vi "20210518_00_ATA_FPGA.vi"() -> ()   [LabVIEW 2018]
doc: "This FPGA VI transfers data samples to the host using a stream. The stream is controlled from the host."
uses:
  FPGA_Controls/FPGA_Enable_Clust.ctl
  FPGA_Controls/FPGA_Scale_Clust.ctl
  FPGA_Controls/FPGA_Probe_Clust.ctl
  <vilib>/Platform/TimedLoop/XDataNode/timing_clust.ctl
  <vilib>/Platform/TimedLoop/XDataNode/nitl_modes.ctl
  <vilib>/Platform/TimedLoop/XDataNode/wakeup.ctl
  FPGA_Controls/FilterStageEnum.ctl
  FPGA_Controls/FPGA_Shift_Enable.ctl
  <vilib>/rvi/Analysis/measure/FFT/simModelSupport/niFPGA FFT Outside SCTL Sim Properties.ctl
  <vilib>/rvi/Analysis/measure/FFT/simModelSupport/niFPGA FFT Sim Types.ctl
  <vilib>/rvi/Analysis/measure/FFT/simModelSupport/niFpgaFFTSimArithmeticProperties.ctl
  <vilib>/rvi/Analysis/measure/FFT/simModelSupport/niFpgaFFTSimDfxp.ctl
  <vilib>/fxp/LVFixedPointQuantizationPolicyTypeDef.ctl
  <vilib>/rvi/Emulation/niFpgaGetClockAttributes.vi
  <vilib>/rvi/Emulation/niFpgaSctlEmulationGetInTimedLoop.vi
  <vilib>/rvi/Emulation/niFpgaEmulationReportErrorSimple.vi
  <vilib>/rvi/eio/common/nirviEmuTemplateMethod_errors.vi
  <vilib>/rvi/Emulation/niFpgaCriticalErrorInLSC.vi
  <vilib>/rvi/DataTransferAndStorage/Container/Common/niFpgaContainerGetUniqueNameForEmu.vi
  <vilib>/rvi/DataTransferAndStorage/Container/Common/niFpgaContainerSetEmuInfo.vi
  <vilib>/rvi/eio/common/nirviEmuReportErrorAndStop.vi
  <vilib>/rvi/DataTransferAndStorage/Container/Common/niFpgaContainerExecOnDevCompGetState.vi
  <vilib>/rvi/Emulation/niFpgaEmulationIsFPGAContextNoSignature.vi
  <vilib>/rvi/Emulation/niFpgaProcessEmulError.vi
  <vilib>/rvi/errors/nirviReportUnexpectedCaseInternalError (U32).vi
  <vilib>/rvi/Memory/Memory_Emulation/niFpgaMemoryEmulationCacheClearOnFirstRun.vi
  <vilib>/rvi/Memory/Memory_Emulation/nirvimemoryEmulationManagerCache_MakeExclusive.vi
  <vilib>/rvi/Memory/Memory_Emulation/niFpgaMemoryEmulationValidateCache.vi
  <vilib>/rvi/Memory/Memory_Emulation/nirvimemoryEmulationManagerCache_InsertValue.vi
  <vilib>/Utility/error.llb/Clear Errors.vi
  <vilib>/rvi/Memory/Memory_Emulation/nirvimemoryEmulationManagerCache_ReleaseExclusive.vi
  <vilib>/rvi/Memory/Memory_Emulation/nirvimemoryEmulationManagerCache_GetValue.vi
  <vilib>/rvi/Memory/Memory_Emulation/nirvimemoryEmulationManagerCache_SetValue.vi
  <vilib>/rvi/Emulation/niFpgaSctlEmulationResourceMgr.vi
  <vilib>/rvi/errors/niFpgaSetErrorForExecOnDevCompSimple.vi
  <vilib>/rvi/FIFO/Fifo_Resource/nirvififoEmulationSetSize.vi
  <vilib>/rvi/FIFO/Fifo_Resource/nirviFifoEmulationQueueMgr.vi
  <instcachedir>/0/nirviFifoEmulationQueueMgr_E5CAEC123FF24DC58D834DCA3CDAA9B5.lvgen/nirviFifoEmulationQueueMgr_E5CAEC123FF24DC58D834DCA3CDAA9B5_000.vi
  <vilib>/rvi/FIFO/Fifo_Resource/nirvififoEmulationCreateLock.vi
  <vilib>/rvi/FIFO/Fifo_Resource/nirvififoEmulationObtainLock.vi
  <vilib>/rvi/FIFO/Fifo_Resource/nirvififoEmulationReleaseLock.vi
  <vilib>/rvi/occurrence/nirviWaitOnOccurrenceBase.vi
  <vilib>/rvi/errors/nirviReportUnexpectedCaseInternalError.vi
  <vilib>/rvi/Analysis/measure/FFT/simModelSupport/niFpgaFFTSimModelOutsideSCTLCore.vi
  <instrlib>/_niInstr/Basic Elements/v1/FPGA/Private/Count Up U16.vi
  <vilib>/rvi/interface/RandomDataEmulation/nirviRandomDataMultiElementFPGAFIFO.vi
  <instcachedir>/0/nirviRandomDataMultiElementFPGAFIFO_6740B454F3C245F78F76ED91F73FD8DB.lvgen/nirviRandomDataMultiElementFPGAFIFO_6740B454F3C245F78F76ED91F73FD8DB_001.vi
  <vilib>/rvi/interface/RandomDataEmulation/niFpgaRandomDataHandleErrors.vi
  <instrlib>/_niInstr/Basic Elements/v1/FPGA/Private/Count Up U32.vi
  <vilib>/rvi/FIFO/Fifo_Resource/nirvififoEmulationDetermineInputValidOut.vi
  <instrlib>/_niInstr/Basic Elements/v1/FPGA/Private/Count Up U8.vi
  <instcachedir>/0/nirviRandomDataMultiElementFPGAFIFO_6740B454F3C245F78F76ED91F73FD8DB.lvgen/nirviRandomDataMultiElementFPGAFIFO_6740B454F3C245F78F76ED91F73FD8DB_000.vi
  <vilib>/eio/EIONode/EIONode.xnode
  <vilib>/Platform/TimedLoop/XDataNode/XDataNode.xnode
  <vilib>/rvi/LocalResourceManager/LocalResourceManager.xnode
  <vilib>/rvi/DataTransferAndStorage/Container/XNode/niFpgaContainer.xnode
  <vilib>/rvi/Memory/Memory_Emulation/niFpgaMemoryEmulationRefIn.vi
  <vilib>/rvi/FIFO/Fifo_Resource/nirvififoEmulationRead.vi
  <vilib>/rvi/Analysis/measure/FFT/XNode/niFpgaFFT.xnode
  <vilib>/rvi/FXPMathLib/FxpMul/XNode/nifxpmath_Multiplier.xnode
  <vilib>/rvi/FXPMathLib/FxpAdd/XNode/nifxpmath_Add.xnode
  <vilib>/rvi/interface/RandomDataEmulation/nirviRandomDataFpgaMultiElementTemplate.vi
  <vilib>/rvi/FXPMathLib/FxpInterpret/XNode/nifxpmath_Interpret.xnode
  <vilib>/rvi/FIFO/Fifo_Resource/niFpgaFifoEmulationRefIn.vi
  <vilib>/Platform/TimedLoop/XDataNode/XDNodeRunTimeDep.lvlib
  <instrlib>/_niInstr/Basic Elements/v1/FPGA/niInstr Basic Elements v1 FPGA.lvlib
  <vilib>/rvi/FXPMathLib/sim/FxpSim.dll
panel:
  out "5_Seconds_Elapsed":bool
  in  "AllData_EvenInvalid":bool
  out "ValidPostShift":bool
  out "ValidPreShift":bool
  out "ValidScaleMeas":bool
  out "WritingToFIFO?":bool
  out "AI0_Unshifted_Index":u32
  out "AI0_Co_Beac_Q_Index":fxp<+/-,24,1>
  out "AI0_Co_I_Index":fxp<+/-,24,1>
  out "MaxMeas":fxp<+/-,24,1>
  in  "Ramp?":bool
  out "AI1_Over":bool
  out "AI0_Over":bool
  in  "Simulate?":bool
  out "Chan1_Beac_QProbe":T1
  out "Chan1_Beac_IProbe":T1
  out "Chan1_Cal_QProbe":T1
  out "Chan0_Beac_QProbe":T1
  out "Chan0_Beac_IProbe":T1
  out "Chan0_Cal_QProbe":T1
  out "NoiseFloorFFT_LoopCount 2":i32
  out "ReceiverTimed Out 2":bool
  out "SuccessiveIndeces 2":u16[](array[numeric])
  in  "#Avg 2":u16=1
  in  "ScaleMeasurement 2":fxp<+/-,16,1>
  in  "Scale_Step1_2":fxp<+/-,17,17>
  in  "EnableStep1_2":bool
  out "Probe 2_2":fxp<+/-,16,16>
  out "Probe 3_2":fxp<+/-,16,1>
  out "Probe 5_2":fxp<+/-,16,2>
  out "Probe 7_2":fxp<+/-,18,1>
  in  "Scale_NoiseFloor 2":fxp<+/-,30,30>
  out "Probe 21_2":fxp<+/-,24,5>
  out "Probe 22_2":fxp<+/-,54,35>
  out "Probe 23_2":fxp<+/-,54,1>
  out "Probe 24_2":fxp<+/-,16,1>
  in  "Offset 2":fxp<+/-,16,16>
  in  "Scale 2":T2={"Scale_Step4"=1.0, "Scale_Step5"=1.0, "Scale_Step6"=1.0, "Scale_Step7"=1.0}
  in  "Enable 2":T3
  in  "FreqShiftCal 2":fxp<+/-,48,0> format="%#.48g"
  out "Chan1_Cal_IProbe":T1
  in  "FreqShiftBeac 2":fxp<+/-,48,0> format="%#.48g"
  out "NoiseFloorFIFOTimeOut 2":bool
  out "Sends 2":u32
  in  "SampleCountReset 2":u32=125000000
  out "Probe 1_2":i16
  out "Probe Offsetd 2":fxp<+/-,16,16>
  out "Probe Offsetd":fxp<+/-,16,16>
  in  "Sample Clock Commit":bool
  in  "Sample Clock Select":u8
  out "SPI Idle":bool
  out "Configuration Error":bool
  out "Synthesizer Locked":bool
  out "Probe 1":i16
  in  "#Avg":u16=1
  in  "SampleCountReset":u32=125000000
  out "ReceiverTimed Out":bool
  out "Sends":u32
  out "SuccessiveIndeces":u16[](array[numeric])
  out "NoiseFloorFFT_LoopCount":i32
  out "NoiseFloorFIFOTimeOut":bool
  in  "FreqShiftBeac":fxp<+/-,48,0> format="%#.48g"
  out "AI0_Cal_IProbe":T1
  in  "Scale":T2={"Scale_Step4"=1.0, "Scale_Step5"=1.0, "Scale_Step6"=1.0, "Scale_Step7"=1.0}
  in  "Enable":T3
  in  "Offset":fxp<+/-,16,16>
  out "Probe 24":fxp<+/-,16,1>
  out "Probe 23":fxp<+/-,54,1>
  out "Probe 22":fxp<+/-,54,35>
  out "Probe 21":fxp<+/-,24,5>
  in  "Scale_NoiseFloor":fxp<+/-,30,30>
  out "Probe 7":fxp<+/-,18,1>
  out "Probe 5":fxp<+/-,16,2>
  out "Probe 3":fxp<+/-,16,1>
  out "Probe 2":fxp<+/-,16,16>
  in  "EnableStep1":bool
  in  "Scale_Step1":fxp<+/-,17,17>
  in  "ScaleMeasurement":fxp<+/-,16,1>
  in  "FreqShiftCal":fxp<+/-,48,0> format="%#.48g"
  out "IO Module\\Initialization Done":bool
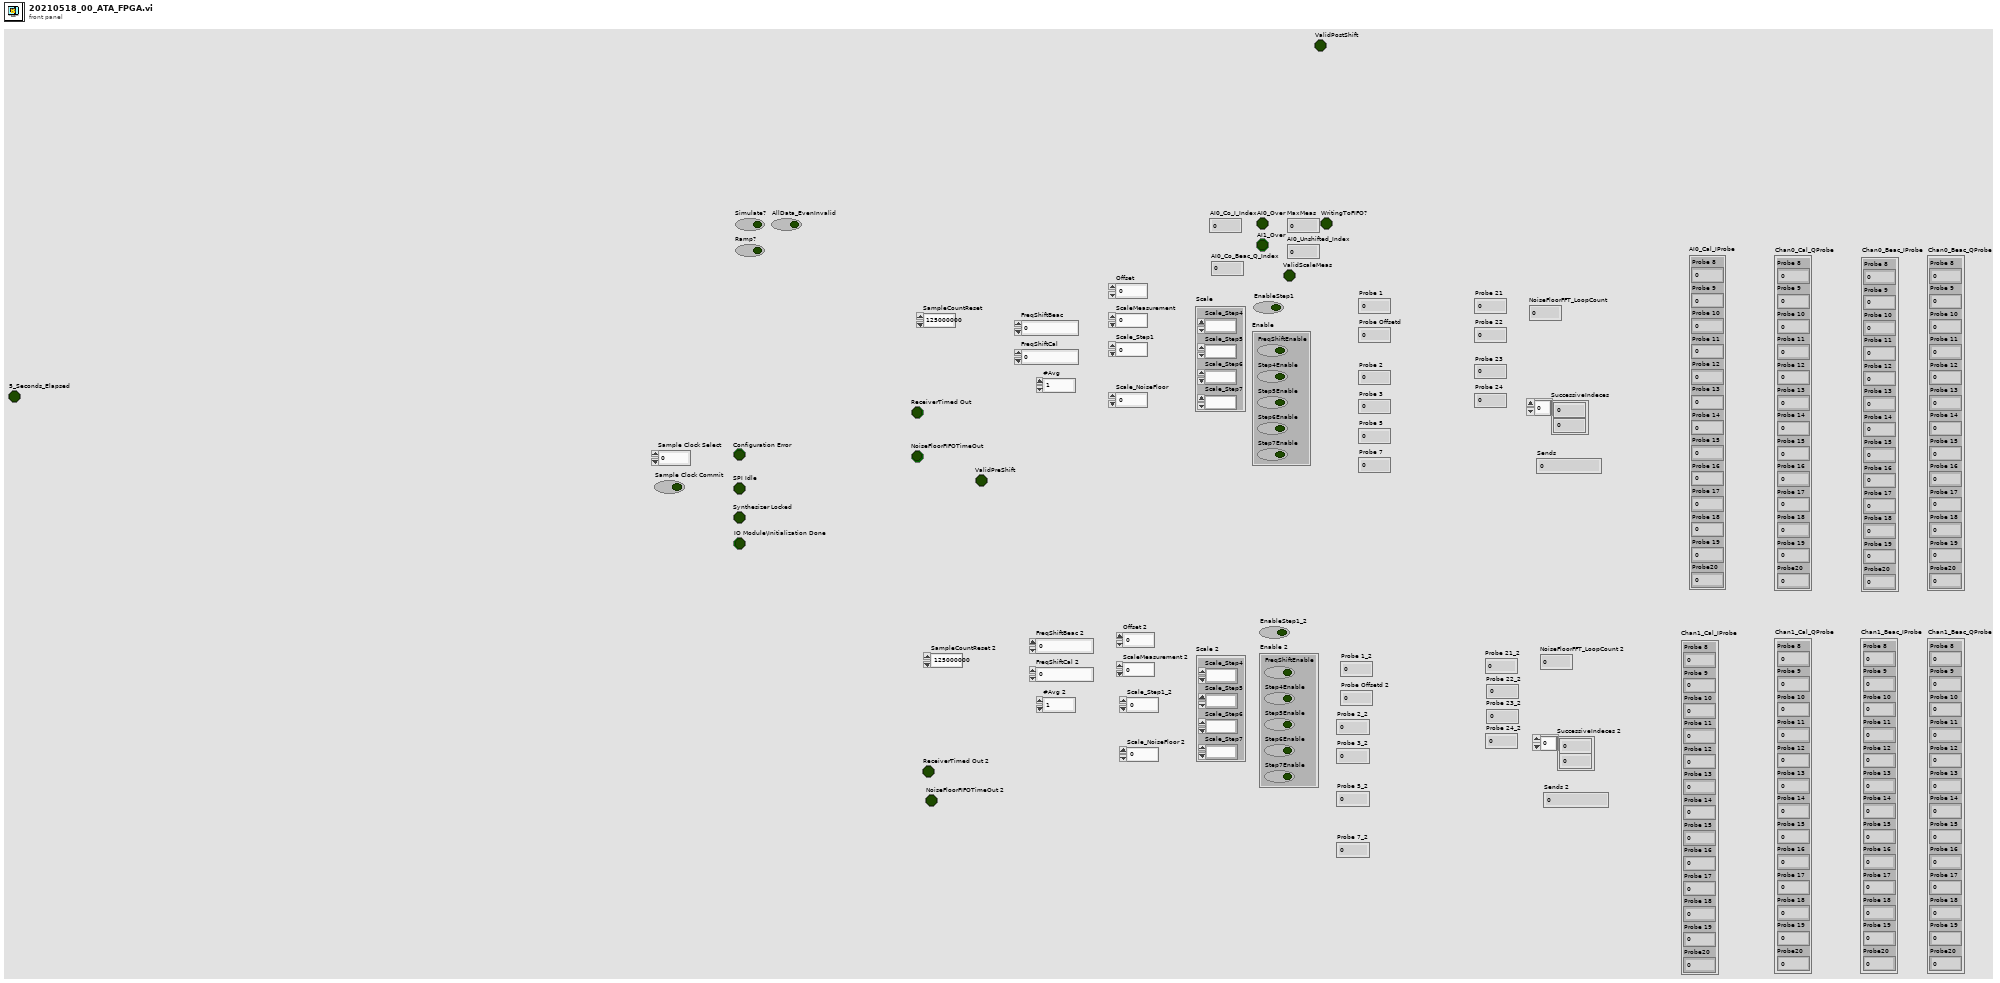
[diagram p1: front panel]
types:
  T1 = typedef "FPGA_Probe_Clust.ctl" = cluster{"Probe 8":fxp<+/-,18,1>, "Probe 9":fxp<+/-,24,1>, "Probe 10":fxp<+/-,24,1>, "Probe 11":fxp<+/-,24,1>, "Probe 12":fxp<+/-,47,24>, "Probe 13":fxp<+/-,24,1>, "Probe 14":fxp<+/-,25,2>, "Probe 15":fxp<+/-,48,25>, "Probe 16":fxp<+/-,24,1>, "Probe 17":fxp<+/-,25,2>, "Probe 18":fxp<+/-,48,25>, "Probe 19":fxp<+/-,24,1>, "Probe20":fxp<+/-,24,1>}
  T2 = typedef "FPGA_Scale_Clust.ctl" = cluster{"Scale_Step4":fxp<+/-,23,23>, "Scale_Step5":fxp<+/-,23,23>, "Scale_Step6":fxp<+/-,23,23>, "Scale_Step7":fxp<+/-,23,23>}
  T3 = typedef "FPGA_Enable_Clust.ctl" = cluster{"FreqShiftEnable":bool, "Step4Enable":bool, "Step5Enable":bool, "Step6Enable":bool, "Step7Enable":bool}
  T4 = typedef "XDNodeRunTimeDep.lvlib/timing_clust.ctl" = cluster{"Expected End [f-1]":u64, "Actual End [f-1]":u64, "Finished Late? [f-1]":bool, "Expected End [i-1]":u64, "Actual End [i-1]":u64, "Finished Late? [i-1]":bool, "Expected Start [i]":u64, "Actual Start [i]":u64, "Expected Start [f]":u64, "Actual Start [f]":u64, "Source Name":string, "Structure Name":string, "Period":i64, "Deadline":i64, "Offset":i64, "Start":i64, "Priority":i32, "Timeout":i32, "Mode":T5, "Wakeup Reason":T6, "Error":errorcluster, "Source Type":string, "Secondary Source Type":string, "Global End Time":u64, "Global Start Time":u64, "Frame Duration":u64, "Iteration Duration":u64, "Assigned CPU":i32, "I/O Scan Engine Mode":u32}
  T5 = typedef "XDNodeRunTimeDep.lvlib/nitl_modes.ctl" = enum32{"No Change", "Process missed periods, maintain original phase", "Discard missed periods, maintain original phase", "Process missed periods, ignore original phase", "Discard missed periods, ignore original phase"}
  T6 = typedef "XDNodeRunTimeDep.lvlib/wakeup.ctl" = enum32{"Normal", "Aborted", "Asynchronous wakeup", "Timing source error", "Timed loop error", "Timeout"}
  T7 = typedef "FPGA_Shift_Enable.ctl" = cluster{"EnableFIFO":bool, "EnableStages":T3}
  T8 = typedef "FilterStageEnum.ctl" = enum16{"Digitiz0", "Digitiz1", "ScaleMeas", "Scale1", "Scale4", "Scale5", "Scale6", "Scale7"}
  T9 = typedef "FPGA_ShiftOutput.ctl" = cluster{"Index":fxp<+/-,24,1>, "output valid":bool, "Data out":fxp<+/-,24,1>, "Probe":T1}
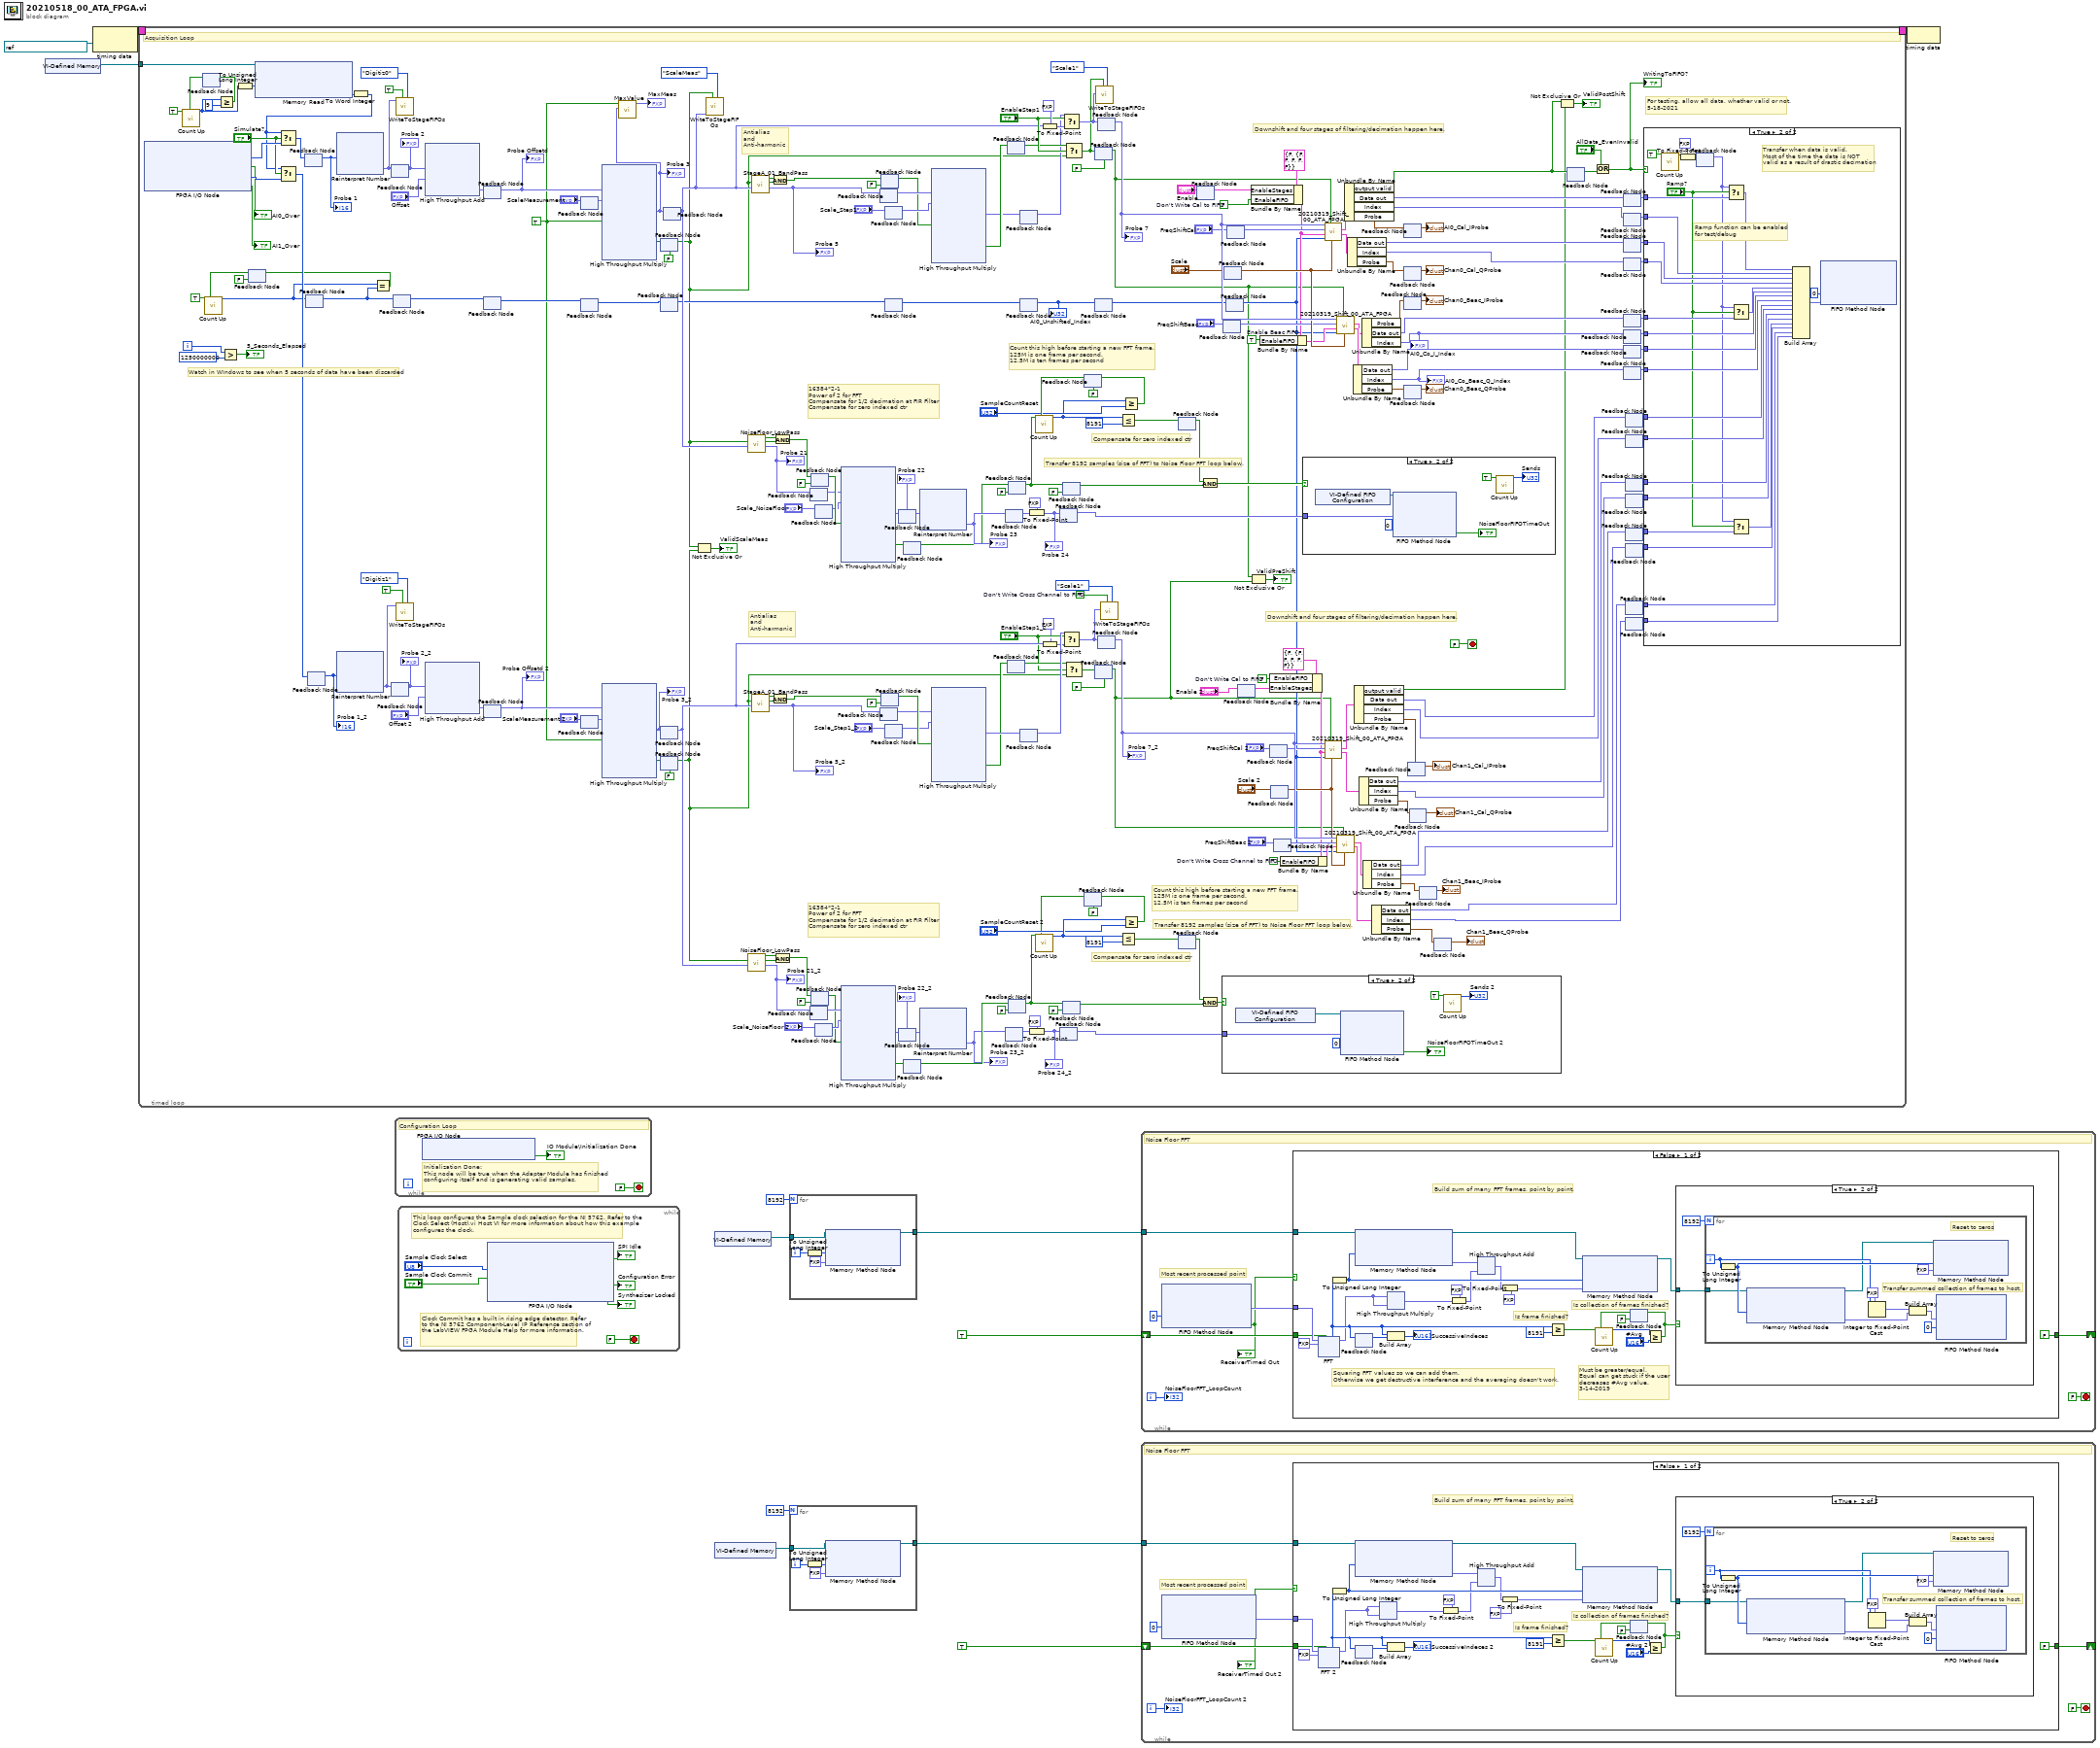
[diagram p0: block diagram]
diagram:
  n1 = xnode "VI-Defined Memory"() -> ("Memory Out"=w1:refnum<k21>)
  n2 = node-c288(refnum<k21> "IO Module\\Data Clock" ("Source Name")) -> (w12:T4)
  n3 = timed-loop {
    timing: w12 -> [_]
    timing-out: [_] -> w11
    tunnel: w1 -> [w123]
    i -> [w13]
    stop <- FALSE stop-if-true
    w74 = FALSE  # Don't Write Cal to FIFO
    w71 = TRUE  # Enable Beac FIFO
    w100 = FALSE  # Don't Write Cross Channel to FIFO
    w64 = FALSE  # Don't Write Cross Channel to FIFO
    w66 = FALSE  # Don't Write Cal to FIFO
    w18 = TRUE ("input valid")
    # "For testing, allow all data, whether valid or not.\n5-18-2021"
    # "Watch in WIndows to see when 5 seconds of data have been discarded"
    # "Downshift and four stages of filtering/decimation happen here."
    # "Downshift and four stages of filtering/decimation happen here."
    # "Antialias\nand\nAnti-harmonic"
    # "Compensate for zero indexed ctr"
    # "16384*2-1\nPower of 2 for FFT\nCompensate for 1/2 decimation at FIR Filter\nCompensate for zero indexed ctr"
    # "Transfer 8192 samples (size of FFT) to Noise Floor FFT loop below."
    # "Count this high before starting a new FFT frame.\n125M is one frame per second.\n12.5M is ten frames per second"
    # "Antialias\nand\nAnti-harmonic"
    # "Compensate for zero indexed ctr"
    # "16384*2-1\nPower of 2 for FFT\nCompensate for 1/2 decimation at FIR Filter\nCompensate for zero indexed ctr"
    # "Transfer 8192 samples (size of FFT) to Noise Floor FFT loop below."
    # "Count this high before starting a new FFT frame.\n125M is one frame per second.\n12.5M is ten frames per second"
    # "Acquisition Loop"
    n4 = xnode "FPGA I/O Node"() -> ("IO Module\\AI 0 Data"=w122:i16, "IO Module\\AI 0 Over Range"=→"AI0_Over":bool, "IO Module\\AI 1 Data"=w117:i16, "IO Module\\AI 1 Over Range"=→"AI1_Over":bool)  [unwired: 4 in, 4 out]
    n5 = feedback #1() -> (w124:bool)  [unwired: 1 in]
    n6 = call-poly <instrlib>:"Count Up.vi"("increment"=TRUE, "reset"=w124) -> ("count out"=w127:u8)  [unwired: 13 in]
    n7 = Greater Or Equal?(x=w127, y=u8 9) -> (x >= y?=w125:bool)
    n8 = feedback-in #1(w125) -> ()
    n9 = Greater?(x=w13, y=1250000000) -> (0:→"5_Seconds_Elapsed":bool)
    n10 = To Unsigned Long Integer(number=w127) -> (unsigned 32bit integer=w129:u32)
    n11 = feedback #2(FALSE) -> (w50:bool)
    n12 = call-poly <instrlib>:"Count Up.vi"("increment"=TRUE, "reset"=w50) -> ("count out"=w48:u32)  [unwired: 13 in]
    n13 = xnode ("Memory Read")("Address"=w129, "Memory In"=w123) -> ("Data"=w120:i8)  [unwired: 1 out]
    n14 = feedback #3() -> (w223:i16)  [unwired: 1 in]
    "Probe 1" <- w223
    n15 = feedback #4() -> (w47:u32)  [unwired: 1 in]
    n16 = feedback-in #4(w48) -> ()
    n17 = feedback #5() -> (w205:i16)  [unwired: 1 in]
    "Probe 1_2" <- w205
    n18 = xnode "Reinterpret Number"("x"=w223) -> ("y"=w104:fxp<+/-,16,16>)
    n19 = xnode "Reinterpret Number"("x"=w205) -> ("y"=w103:fxp<+/-,16,16>)
    n20 = To Word Integer(number=w120) -> (16bit integer=w116:i16)
    n21 = Select(t=w116, s="Simulate?", f=w122) -> (s? t:f=w121:i16)
    n22 = Select(t=w116, s="Simulate?", f=w117) -> (s? t:f=w118:i16)
    n23 = feedback-in #3(w121) -> ()
    n24 = feedback-in #5(w118) -> ()
    n25 = Equal?(x=w48, y=w47) -> (x = y?=w51:bool)
    n26 = feedback-in #2(w51) -> ()
    n27 = feedback #6() -> (w236:fxp<+/-,16,16>)  [unwired: 1 in]
    "Probe 2" <- w236
    n28 = feedback-in #6(w104) -> ()
    n29 = feedback #7() -> (w198:fxp<+/-,16,16>)  [unwired: 1 in]
    "Probe 2_2" <- w198
    n30 = feedback-in #7(w103) -> ()
    n31 = feedback #8() -> (w52:u32)  [unwired: 1 in]
    n32 = feedback-in #8(w47) -> ()
    n33 = call "WriteToStageFIFOs.vi"("Stage"=FilterStageEnum."Digitiz0", "Enable"=TRUE, "Digitiz"=w104) -> ()  [unwired: 9 in]
    n34 = call "WriteToStageFIFOs.vi"("Stage"=FilterStageEnum."Digitiz1", "Enable"=TRUE, "Digitiz"=w103) -> ()  [unwired: 9 in]
    n35 = xnode ("High Throughput Add")("x"=w236, "y"="Offset") -> ("x+y"=w235:fxp<+/-,16,16>)
    n36 = xnode ("High Throughput Add")("x"=w198, "y"="Offset 2") -> ("x+y"=w106:fxp<+/-,16,16>)
    n37 = feedback #9() -> (w113:fxp<+/-,16,16>)  [unwired: 1 in]
    "Probe Offsetd" <- w113
    n38 = feedback-in #9(w235) -> ()
    n39 = feedback #10() -> (w94:u32)  [unwired: 1 in]
    n40 = feedback-in #10(w52) -> ()
    n41 = feedback #11() -> (w105:fxp<+/-,16,16>)  [unwired: 1 in]
    "Probe Offsetd 2" <- w105
    n42 = feedback-in #11(w106) -> ()
    n43 = feedback #12() -> (w264:fxp<+/-,16,1>)  [unwired: 1 in]
    n44 = feedback-in #12("ScaleMeasurement") -> ()
    n45 = feedback #13() -> (w93:u32)  [unwired: 1 in]
    n46 = feedback-in #13(w94) -> ()
    n47 = feedback #14() -> (w169:fxp<+/-,16,1>)  [unwired: 1 in]
    n48 = feedback-in #14("ScaleMeasurement 2") -> ()
    n49 = xnode ("High Throughput Multiply")("x"=w113, "y"=w264, "input valid"=w18) -> ("x*y"=w112:fxp<+/-,16,1>, "output valid"=w238:bool)  [unwired: 1 in, 1 out]
    "Probe 3" <- w112
    n50 = xnode ("High Throughput Multiply")("x"=w105, "y"=w169, "input valid"=w18) -> ("x*y"=w166:fxp<+/-,16,1>, "output valid"=w196:bool)  [unwired: 1 in, 1 out]
    "Probe 3_2" <- w166
    n51 = call "MaxValue.vi"("NewValue"=w112, "DataValid"=w18) -> ("Max"=→"MaxMeas":fxp<+/-,24,1>)  [unwired: 9 in]
    n52 = feedback #15(FALSE ("output valid")) -> (w29:bool)
    n53 = feedback-in #15(w238) -> ()
    n54 = feedback #16() -> (w92:u32)  [unwired: 1 in]
    n55 = feedback-in #16(w93) -> ()
    n56 = feedback #17() -> (w208:fxp<+/-,16,1>)  [unwired: 1 in]
    n57 = feedback-in #17(w166) -> ()
    n58 = feedback #18(FALSE ("output valid")) -> (w28:bool)
    n59 = feedback-in #18(w196) -> ()
    n60 = feedback #19() -> (w96:fxp<+/-,16,1>)  [unwired: 1 in]
    n61 = feedback-in #19(w112) -> ()
    n62 = Not Exclusive Or(1:w28, 2:w29) -> (0:→"ValidScaleMeas":bool)
    n63 = call "WriteToStageFIFOs.vi"("Stage"=FilterStageEnum."ScaleMeas", "Enable"=w29, "ScaleMeas"=w96) -> ()  [unwired: 9 in]
    n64 = call "NoiseFloor_LowPass.vi"("s_axis_data_tdata"=w96, "s_axis_data_tvalid"=w29) -> ("m_axis_data_tdata"=w248:fxp<+/-,24,5>, "m_axis_data_tvalid"=w255:bool, "s_axis_data_tready"=w256:bool)  [unwired: 7 in]
    "Probe 21" <- w248
    n65 = call "NoiseFloor_LowPass.vi"("s_axis_data_tdata"=w208, "s_axis_data_tvalid"=w28) -> ("m_axis_data_tdata"=w186:fxp<+/-,24,5>, "m_axis_data_tvalid"=w179:bool, "s_axis_data_tready"=w178:bool)  [unwired: 7 in]
    "Probe 21_2" <- w186
    n66 = call "StageA_01_BandPass.vi"("s_axis_data_tdata"=w96, "s_axis_data_tvalid"=w29) -> ("m_axis_data_tdata"=w220:fxp<+/-,16,2>, "m_axis_data_tvalid"=w269:bool, "s_axis_data_tready"=w270:bool)  [unwired: 7 in]
    "Probe 5" <- w220
    n67 = call "StageA_01_BandPass.vi"("s_axis_data_tdata"=w208, "s_axis_data_tvalid"=w28) -> ("m_axis_data_tdata"=w209:fxp<+/-,16,2>, "m_axis_data_tvalid"=w163:bool, "s_axis_data_tready"=w162:bool)  [unwired: 7 in]
    "Probe 5_2" <- w209
    n68 = And(x=w270, y=w269) -> (x .and. y?=w221:bool)
    n69 = And(x=w162, y=w163) -> (x .and. y?=w207:bool)
    n70 = And(x=w256, y=w255) -> (x .and. y?=w247:bool)
    n71 = And(x=w178, y=w179) -> (x .and. y?=w187:bool)
    n72 = feedback #20() -> (w249:fxp<+/-,24,5>)  [unwired: 1 in]
    n73 = feedback-in #20(w248) -> ()
    n74 = feedback #21() -> (w185:fxp<+/-,24,5>)  [unwired: 1 in]
    n75 = feedback-in #21(w186) -> ()
    n76 = feedback #22(FALSE ("s_axis_data_tvalid")) -> (w252:bool)
    n77 = feedback-in #22(w247) -> ()
    n78 = feedback #23(FALSE ("s_axis_data_tvalid")) -> (w182:bool)
    n79 = feedback-in #23(w187) -> ()
    n80 = feedback #24() -> (w251:fxp<+/-,30,30>)  [unwired: 1 in]
    n81 = feedback-in #24("Scale_NoiseFloor") -> ()
    n82 = feedback #25() -> (w183:fxp<+/-,30,30>)  [unwired: 1 in]
    n83 = feedback-in #25("Scale_NoiseFloor 2") -> ()
    n84 = xnode ("High Throughput Multiply")("x"=w249, "y"=w251, "input valid"=w252) -> ("x*y"=w244:fxp<+/-,54,35>, "output valid"=w241:bool)  [unwired: 1 in, 1 out]
    "Probe 22" <- w244
    n85 = xnode ("High Throughput Multiply")("x"=w185, "y"=w183, "input valid"=w182) -> ("x*y"=w190:fxp<+/-,54,35>, "output valid"=w193:bool)  [unwired: 1 in, 1 out]
    "Probe 22_2" <- w190
    n86 = feedback #26() -> (w266:fxp<+/-,16,2>)  [unwired: 1 in]
    n87 = feedback-in #26(w220) -> ()
    n88 = feedback #27() -> (w167:fxp<+/-,16,2>)  [unwired: 1 in]
    n89 = feedback-in #27(w209) -> ()
    n90 = feedback #28(FALSE ("s_axis_data_tvalid")) -> (w262:bool)
    n91 = feedback-in #28(w221) -> ()
    n92 = feedback #29(FALSE ("s_axis_data_tvalid")) -> (w171:bool)
    n93 = feedback-in #29(w207) -> ()
    n94 = feedback #30() -> (w263:fxp<+/-,17,17>)  [unwired: 1 in]
    n95 = feedback-in #30("Scale_Step1") -> ()
    n96 = feedback #31() -> (w91:u32)  [unwired: 1 in]
    n97 = feedback-in #31(w92) -> ()
    n98 = feedback #32() -> (w170:fxp<+/-,17,17>)  [unwired: 1 in]
    n99 = feedback-in #32("Scale_Step1_2") -> ()
    n100 = feedback #33() -> (w243:fxp<+/-,54,35>)  [unwired: 1 in]
    n101 = feedback-in #33(w244) -> ()
    n102 = feedback #34() -> (w191:fxp<+/-,54,35>)  [unwired: 1 in]
    n103 = feedback-in #34(w190) -> ()
    n104 = feedback #35() -> (w240:bool)  [unwired: 1 in]
    n105 = feedback-in #35(w241) -> ()
    n106 = feedback #36() -> (w194:bool)  [unwired: 1 in]
    n107 = feedback-in #36(w193) -> ()
    n108 = xnode "Reinterpret Number"("x"=w243) -> ("y"=w242:fxp<+/-,54,1>)
    "Probe 23" <- w242
    n109 = xnode "Reinterpret Number"("x"=w191) -> ("y"=w192:fxp<+/-,54,1>)
    "Probe 23_2" <- w192
    n110 = xnode ("High Throughput Multiply")("x"=w266, "y"=w263, "input valid"=w262) -> ("x*y"=w217:fxp<+/-,18,1>, "output valid"=w219:bool)  [unwired: 1 in, 1 out]
    n111 = xnode ("High Throughput Multiply")("x"=w167, "y"=w170, "input valid"=w171) -> ("x*y"=w212:fxp<+/-,18,1>, "output valid"=w210:bool)  [unwired: 1 in, 1 out]
    n112 = feedback #37() -> (w245:fxp<+/-,54,1>)  [unwired: 1 in]
    n113 = feedback-in #37(w242) -> ()
    n114 = feedback #38() -> (w189:fxp<+/-,54,1>)  [unwired: 1 in]
    n115 = feedback-in #38(w192) -> ()
    n116 = feedback #39() -> (w218:bool)  [unwired: 1 in]
    n117 = feedback-in #39(w219) -> ()
    n118 = feedback #40() -> (w211:bool)  [unwired: 1 in]
    n119 = feedback-in #40(w210) -> ()
    n120 = feedback #41(FALSE ("output valid")) -> (w234:bool)
    n121 = feedback-in #41(w240) -> ()
    n122 = feedback #42(FALSE ("output valid")) -> (w199:bool)
    n123 = feedback-in #42(w194) -> ()
    n124 = feedback #43() -> (w216:fxp<+/-,18,1>)  [unwired: 1 in]
    n125 = feedback-in #43(w217) -> ()
    n126 = feedback #44() -> (w90:u32)  [unwired: 1 in]
    "AI0_Unshifted_Index" <- w90
    n127 = feedback-in #44(w91) -> ()
    n128 = feedback #45() -> (w213:fxp<+/-,18,1>)  [unwired: 1 in]
    n129 = feedback-in #45(w212) -> ()
    n130 = To Fixed-Point(fixed-point type=fxp<+/-,16,1> 0.0, number=w245) -> (fixed-point=w224:fxp<+/-,16,1>)
    "Probe 24" <- w224
    n131 = To Fixed-Point(fixed-point type=fxp<+/-,16,1> 0.0, number=w189) -> (fixed-point=w204:fxp<+/-,16,1>)
    "Probe 24_2" <- w204
    n132 = To Fixed-Point(fixed-point type=fxp<+/-,18,1> 0.0, number=w96) -> (fixed-point=w260:fxp<+/-,18,1>)
    n133 = To Fixed-Point(fixed-point type=fxp<+/-,18,1> 0.0, number=w208) -> (fixed-point=w174:fxp<+/-,18,1>)
    n134 = feedback #46() -> (w225:fxp<+/-,16,1>)  [unwired: 1 in]
    n135 = feedback-in #46(w224) -> ()
    n136 = feedback #47() -> (w203:fxp<+/-,16,1>)  [unwired: 1 in]
    n137 = feedback-in #47(w204) -> ()
    n138 = feedback #48(FALSE ("output valid")) -> (w232:bool)
    n139 = feedback-in #48(w234) -> ()
    n140 = feedback #49(FALSE ("output valid")) -> (w201:bool)
    n141 = feedback-in #49(w199) -> ()
    n142 = Select(t=w216, s="EnableStep1", f=w260) -> (s? t:f=w108:fxp<+/-,18,1>)
    n143 = Select(t=w213, s="EnableStep1_2", f=w174) -> (s? t:f=w101:fxp<+/-,18,1>)
    n144 = Select(t=w218, s="EnableStep1", f=w29) -> (s? t:f=w95:bool)
    n145 = Select(t=w211, s="EnableStep1_2", f=w28) -> (s? t:f=w172:bool)
    n146 = feedback #50(FALSE ("reset")) -> (w275:bool)
    n147 = call-poly <instrlib>:"Count Up.vi"("increment"=w234, "reset"=w275) -> ("count out"=w268:u32)  [unwired: 13 in]
    n148 = feedback #51(FALSE ("reset")) -> (w157:bool)
    n149 = call-poly <instrlib>:"Count Up.vi"("increment"=w199, "reset"=w157) -> ("count out"=w164:u32)  [unwired: 13 in]
    n150 = feedback #52(FALSE ("s_axis_data_tvalid")) -> (w25:bool)
    n151 = feedback-in #52(w95) -> ()
    n152 = feedback #53() -> (w89:u32)  [unwired: 1 in]
    n153 = feedback-in #53(w90) -> ()
    n154 = feedback #54(FALSE ("s_axis_data_tvalid")) -> (w24:bool)
    n155 = feedback-in #54(w172) -> ()
    n156 = call "WriteToStageFIFOs.vi"("Stage"=FilterStageEnum."Scale1", "Enable"=w95, "Scale1"=w108) -> ()  [unwired: 9 in]
    n157 = feedback #55() -> (w215:fxp<+/-,18,1>)  [unwired: 1 in]
    "Probe 7" <- w215
    n158 = feedback-in #55(w108) -> ()
    n159 = feedback #56() -> (w214:fxp<+/-,18,1>)  [unwired: 1 in]
    "Probe 7_2" <- w214
    n160 = feedback-in #56(w101) -> ()
    n161 = call "WriteToStageFIFOs.vi"("Stage"=FilterStageEnum."Scale1", "Enable"=w100, "Scale1"=w101) -> ()  [unwired: 9 in]
    n162 = Less Or Equal?(x=w268, y=u32 8191) -> (x <= y?=w276:bool)
    n163 = Less Or Equal?(x=w164, y=u32 8191) -> (x <= y?=w156:bool)
    n164 = Greater Or Equal?(x=w268, y="SampleCountReset") -> (x >= y?=w272:bool)
    n165 = feedback-in #50(w272) -> ()
    n166 = Greater Or Equal?(x=w164, y="SampleCountReset 2") -> (x >= y?=w160:bool)
    n167 = feedback-in #51(w160) -> ()
    n168 = feedback #57() -> (w233:bool)  [unwired: 1 in]
    n169 = feedback-in #57(w276) -> ()
    n170 = feedback #58() -> (w200:bool)  [unwired: 1 in]
    n171 = feedback-in #58(w156) -> ()
    n172 = feedback #59() -> (w75:T3)  [unwired: 1 in]
    n173 = feedback-in #59("Enable") -> ()
    n174 = And(x=w233, y=w232) -> (x .and. y?=w231:bool)
    n175 = And(x=w200, y=w201) -> (x .and. y?=w202:bool)
    n176 = case shown="True" w202 {
      tunnel: w203 -> [_ w282]
      frame False {
      }
      frame True {
        n177 = xnode "VI-Defined FIFO Configuration"() -> ("FIFO Out"=w277:refnum<k21>)
        n178 = xnode ("FIFO Method Node")("Element"=w282, "Timeout"=0, "FIFO In"=w277) -> ("Timed Out?"=→"NoiseFloorFIFOTimeOut 2":bool)  [unwired: 1 out]
        n179 = call-poly <instrlib>:"Count Up.vi"("increment"=TRUE) -> ("count out"=→"Sends 2":u32)  [unwired: 14 in]
      }
    }
    n180 = feedback #60() -> (w142:fxp<+/-,48,0>)  [unwired: 1 in]
    n181 = feedback-in #60("FreqShiftBeac") -> ()
    n182 = feedback #61() -> (w144:T2)  [unwired: 1 in]
    n183 = feedback-in #61("Scale") -> ()
    n184 = feedback #62() -> (w46:u32)  [unwired: 1 in]
    n185 = feedback-in #62(w89) -> ()
    n186 = feedback #63() -> (w140:fxp<+/-,48,0>)  [unwired: 1 in]
    n187 = feedback-in #63("FreqShiftCal") -> ()
    n188 = feedback #64() -> (w19:T3)  [unwired: 1 in]
    n189 = feedback-in #64("Enable 2") -> ()
    n190 = Not Exclusive Or(1:w24, 2:w25) -> (0:→"ValidPreShift":bool)
    n191 = Bundle By Name(cluster=T7 {"EnableFIFO"=FALSE, "EnableStages"={"FreqShiftEnable"=FALSE, "Step4Enable"=FALSE, "Step5Enable"=FALSE, "Step6Enable"=FALSE, "Step7Enable"=FALSE}}, "EnableStages"=w75, "EnableFIFO"=w74) -> (w73:T7)
    n192 = Bundle By Name(cluster=w73, "EnableFIFO"=w71) -> (w72:T7)
    n193 = Bundle By Name(cluster=T7 {"EnableFIFO"=FALSE, "EnableStages"={"FreqShiftEnable"=FALSE, "Step4Enable"=FALSE, "Step5Enable"=FALSE, "Step6Enable"=FALSE, "Step7Enable"=FALSE}}, "EnableFIFO"=w66, "EnableStages"=w19) -> (w62:T7)
    n194 = feedback #65() -> (w138:fxp<+/-,48,0>)  [unwired: 1 in]
    n195 = feedback-in #65("FreqShiftCal 2") -> ()
    n196 = feedback #66() -> (w130:T2)  [unwired: 1 in]
    n197 = feedback-in #66("Scale 2") -> ()
    n198 = feedback #67() -> (w136:fxp<+/-,48,0>)  [unwired: 1 in]
    n199 = feedback-in #67("FreqShiftBeac 2") -> ()
    n200 = Bundle By Name(cluster=w62, "EnableFIFO"=w64) -> (w63:T7)
    n201 = case shown="True" w231 {
      tunnel: w225 -> [_ w288]
      frame False {
      }
      frame True {
        n202 = xnode "VI-Defined FIFO Configuration"() -> ("FIFO Out"=w283:refnum<k21>)
        n203 = xnode ("FIFO Method Node")("Element"=w288, "Timeout"=0, "FIFO In"=w283) -> ("Timed Out?"=→"NoiseFloorFIFOTimeOut":bool)  [unwired: 1 out]
        n204 = call-poly <instrlib>:"Count Up.vi"("increment"=TRUE) -> ("count out"=→"Sends":u32)  [unwired: 14 in]
      }
    }
    n205 = call "20210319_Shift_00_ATA_FPGA.vi"("Scale"=w144, "Input valid"=w25, "Index"=w46, "Enable"=w73, "frequency shift"=w140, "Data in"=w215) -> ("Q Shift Output"=w155:T9, "I Shift Output"=w152:T9)  [unwired: 4 in]
    n206 = call "20210319_Shift_00_ATA_FPGA.vi"("Scale"=w130, "Input valid"=w24, "Index"=w46, "Enable"=w62, "frequency shift"=w138, "Data in"=w214) -> ("Q Shift Output"=w61:T9, "I Shift Output"=w65:T9)  [unwired: 4 in]
    n207 = call "20210319_Shift_00_ATA_FPGA.vi"("Scale"=w144, "Input valid"=w25, "Index"=w46, "Enable"=w72, "frequency shift"=w142, "Data in"=w215) -> ("Q Shift Output"=w229:T9, "I Shift Output"=w149:T9)  [unwired: 4 in]
    n208 = call "20210319_Shift_00_ATA_FPGA.vi"("Scale"=w130, "Input valid"=w24, "Index"=w46, "Enable"=w63, "frequency shift"=w136, "Data in"=w214) -> ("Q Shift Output"=w56:T9, "I Shift Output"=w58:T9)  [unwired: 4 in]
    n209 = Unbundle By Name(w152) -> ("output valid"=w22:bool, "Data out"=w80:fxp<+/-,24,1>, "Index"=w82:fxp<+/-,24,1>, "Probe"=w88:T1)
    n210 = Unbundle By Name(w155) -> ("Data out"=w78:fxp<+/-,24,1>, "Index"=w87:fxp<+/-,24,1>, "Probe"=w68:T1)
    n211 = Unbundle By Name(w229) -> ("Data out"=w85:fxp<+/-,24,1>, "Index"=w54:fxp<+/-,24,1>, "Probe"=w84:T1)
    "AI0_Co_Beac_Q_Index" <- w54
    n212 = Unbundle By Name(w65) -> ("output valid"=w21:bool, "Data out"=w38:fxp<+/-,24,1>, "Index"=w39:fxp<+/-,24,1>, "Probe"=w60:T1)
    n213 = Unbundle By Name(w61) -> ("Data out"=w40:fxp<+/-,24,1>, "Index"=w41:fxp<+/-,24,1>, "Probe"=w59:T1)
    n214 = Unbundle By Name(w149) -> ("Probe"=w86:T1, "Data out"=w83:fxp<+/-,24,1>, "Index"=w70:fxp<+/-,24,1>)
    "AI0_Co_I_Index" <- w70
    n215 = Unbundle By Name(w58) -> ("Data out"=w42:fxp<+/-,24,1>, "Index"=w43:fxp<+/-,24,1>, "Probe"=w57:T1)
    n216 = Unbundle By Name(w56) -> ("Data out"=w44:fxp<+/-,24,1>, "Index"=w45:fxp<+/-,24,1>, "Probe"=w55:T1)
    n217 = feedback #68() -> (→"AI0_Cal_IProbe":T1)  [unwired: 1 in]
    n218 = feedback-in #68(w88) -> ()
    n219 = feedback #69() -> (→"Chan0_Cal_QProbe":T1)  [unwired: 1 in]
    n220 = feedback-in #69(w68) -> ()
    n221 = feedback #70() -> (→"Chan0_Beac_IProbe":T1)  [unwired: 1 in]
    n222 = feedback-in #70(w86) -> ()
    n223 = feedback #71() -> (→"Chan0_Beac_QProbe":T1)  [unwired: 1 in]
    n224 = feedback-in #71(w84) -> ()
    n225 = feedback #72() -> (→"Chan1_Cal_IProbe":T1)  [unwired: 1 in]
    n226 = feedback-in #72(w60) -> ()
    n227 = feedback #73() -> (→"Chan1_Cal_QProbe":T1)  [unwired: 1 in]
    n228 = feedback-in #73(w59) -> ()
    n229 = feedback #74() -> (→"Chan1_Beac_IProbe":T1)  [unwired: 1 in]
    n230 = feedback-in #74(w57) -> ()
    n231 = feedback #75() -> (→"Chan1_Beac_QProbe":T1)  [unwired: 1 in]
    n232 = feedback-in #75(w55) -> ()
    n233 = Not Exclusive Or(1:w21, 2:w22) -> (0:→"ValidPostShift":bool)
    n234 = feedback #76() -> (w226:bool)  [unwired: 1 in]
    n235 = feedback-in #76(w22) -> ()
    n236 = Or(x="AllData_EvenInvalid", y=w226) -> (x .or. y?=w17:bool)
    "WritingToFIFO?" <- w17
    n237 = feedback #77() -> (w227:fxp<+/-,24,1>)  [unwired: 1 in]
    n238 = feedback-in #77(w80) -> ()
    n239 = feedback #78() -> (w81:fxp<+/-,24,1>)  [unwired: 1 in]
    n240 = feedback-in #78(w82) -> ()
    n241 = feedback #79() -> (w77:fxp<+/-,24,1>)  [unwired: 1 in]
    n242 = feedback-in #79(w78) -> ()
    n243 = feedback #80() -> (w153:fxp<+/-,24,1>)  [unwired: 1 in]
    n244 = feedback-in #80(w87) -> ()
    n245 = feedback #81() -> (w154:fxp<+/-,24,1>)  [unwired: 1 in]
    n246 = feedback-in #81(w83) -> ()
    n247 = feedback #82() -> (w69:fxp<+/-,24,1>)  [unwired: 1 in]
    n248 = feedback-in #82(w70) -> ()
    n249 = feedback #83() -> (w228:fxp<+/-,24,1>)  [unwired: 1 in]
    n250 = feedback-in #83(w85) -> ()
    n251 = feedback #84() -> (w79:fxp<+/-,24,1>)  [unwired: 1 in]
    n252 = feedback-in #84(w54) -> ()
    n253 = feedback #85() -> (w37:fxp<+/-,24,1>)  [unwired: 1 in]
    n254 = feedback-in #85(w38) -> ()
    n255 = feedback #86() -> (w36:fxp<+/-,24,1>)  [unwired: 1 in]
    n256 = feedback-in #86(w39) -> ()
    n257 = feedback #87() -> (w35:fxp<+/-,24,1>)  [unwired: 1 in]
    n258 = feedback-in #87(w40) -> ()
    n259 = feedback #88() -> (w34:fxp<+/-,24,1>)  [unwired: 1 in]
    n260 = feedback-in #88(w41) -> ()
    n261 = feedback #89() -> (w33:fxp<+/-,24,1>)  [unwired: 1 in]
    n262 = feedback-in #89(w42) -> ()
    n263 = feedback #90() -> (w32:fxp<+/-,24,1>)  [unwired: 1 in]
    n264 = feedback-in #90(w43) -> ()
    n265 = feedback #91() -> (w31:fxp<+/-,24,1>)  [unwired: 1 in]
    n266 = feedback-in #91(w44) -> ()
    n267 = feedback #92() -> (w30:fxp<+/-,24,1>)  [unwired: 1 in]
    n268 = feedback-in #92(w45) -> ()
    n269 = case shown="True" w17 {
      tunnel: w227 -> [_ w311]
      tunnel: w228 -> [_ w302]
      tunnel: w154 -> [_ w300]
      tunnel: w153 -> [_ w306]
      tunnel: w81 -> [_ w309]
      tunnel: w77 -> [_ w307]
      tunnel: w79 -> [_ w308]
      tunnel: w69 -> [_ w305]
      tunnel: w37 -> [_ w299]
      tunnel: w36 -> [_ w298]
      tunnel: w35 -> [_ w297]
      tunnel: w34 -> [_ w296]
      tunnel: w33 -> [_ w292]
      tunnel: w32 -> [_ w295]
      tunnel: w31 -> [_ w294]
      tunnel: w30 -> [_ w293]
      frame False {
        # "Ready last time?"
      }
      frame True {
        # "Ramp function can be enabled\nfor test/debug"
        # "Transfer when data is valid.\nMost of the time the data is NOT\nvalid as a result of drastic decimation"
        n270 = call-poly <instrlib>:"Count Up.vi"("increment"=TRUE) -> ("count out"=w313:u32)  [unwired: 14 in]
        n271 = To Fixed-Point(fixed-point type=fxp<+/-,24,1> 0.0, number=w313) -> (fixed-point=w312:fxp<+/-,24,1>)
        n272 = feedback-in #93(w312) -> ()
        n273 = feedback #93() -> (w289:fxp<+/-,24,1>)  [unwired: 1 in]
        n274 = Select(t=w289, s="Ramp?", f=w311) -> (s? t:f=w310:fxp<+/-,24,1>)
        n275 = Select(t=w289, s="Ramp?", f=w300) -> (s? t:f=w301:fxp<+/-,24,1>)
        n276 = Select(t=w289, s="Ramp?", f=w292) -> (s? t:f=w290:fxp<+/-,24,1>)
        n277 = Build Array(w310, w309, w307, w306, w301, w305, w302, w308, w299, w298, w297, w296, w290, w295, w294, w293) -> (w304:fxp<+/-,24,1>[])
        n278 = xnode ("FIFO Method Node")("Element"=w304, "Timeout"=0) -> ()  [unwired: 1 in, 2 out]
      }
    }
  }
  n279 = while {
    stop <- FALSE stop-if-true
    # "Initialization Done:\nThis node will be true when the Adapter Module has finished configuring itself and is generating valid samples."
    # "Configuration Loop"
    n280 = xnode "FPGA I/O Node"() -> ("IO Module\\Initialization Done"=→"IO Module\\Initialization Done":bool)  [unwired: 1 in, 1 out]
  }
  n281 = while {
    stop <- FALSE stop-if-true
    # "Clock Commit has a built in rising edge detector. Refer to the NI 5762 Component-Level IP Reference section of the LabVIEW FPGA Module Help for more information."
    # "This loop configures the Sample clock selection for the NI 5762. Refer to the Clock Select (Host).vi Host VI for more information about how this example configures the clock."
    n282 = xnode "FPGA I/O Node"("IO Module\\Sample Clock Select"="Sample Clock Select", "IO Module\\Sample Clock Commit"="Sample Clock Commit") -> ("IO Module\\SPI Idle"=→"SPI Idle":bool, "IO Module\\Configuration Error"=→"Configuration Error":bool, "IO Module\\PLL Locked"=→"Synthesizer Locked":bool)  [unwired: 5 in, 5 out]
  }
  n283 = xnode "VI-Defined Memory"() -> ("Memory Out"=w6:refnum<k21>)
  n284 = xnode "VI-Defined Memory"() -> ("Memory Out"=w5:refnum<k21>)
  n285 = for {
    N: 8192 ("dimension size") -> [_]
    tunnel: [w327] -> w7
    tunnel: w6 -> [w326]
    i -> [w330]
    n286 = To Unsigned Long Integer(number=w330) -> (unsigned 32bit integer=w329:u32)
    n287 = xnode ("Memory Method Node")("Address"=w329, "Data"=fxp<+/-,27,12> 0.0, "Memory In"=w326) -> ("Memory Out"=w327:refnum<k21>)
  }
  n288 = for {
    N: 8192 ("dimension size") -> [_]
    tunnel: [w332] -> w4
    tunnel: w5 -> [w331]
    i -> [w335]
    n289 = To Unsigned Long Integer(number=w335) -> (unsigned 32bit integer=w334:u32)
    n290 = xnode ("Memory Method Node")("Address"=w334, "Data"=fxp<+/-,27,12> 0.0, "Memory In"=w331) -> ("Memory Out"=w332:refnum<k21>)
  }
  n291 = while {
    shift-right: [w338] -> _
    shift-left: TRUE -> [w339]
    tunnel: w7 -> [w336]
    i -> [w340]
    stop <- FALSE stop-if-true
    # "Most recent processed point"
    # "Noise Floor FFT"
    n292 = xnode ("FIFO Method Node")("Timeout"=0) -> ("Element"=w342:fxp<+/-,16,1>, "Timed Out?"=w337:bool)  [unwired: 1 in, 1 out]
    "ReceiverTimed Out" <- w337
    n293 = case shown="False" w337 {
      tunnel: w342 -> [w369 _]
      tunnel: w339 -> [w368 w401]
      tunnel: [FALSE w401] -> w338
      tunnel: w336 -> [w350 _]
      frame False {
        # "Squaring FFT values so we can add them. \nOtherwise we get destructive interference and the averaging doesn't work."
        # "Must be greater/equal.\nEqual can get stuck if the user\ndecreases #Avg value.\n3-14-2019"
        # "Is collection of frames finished?"
        # "Is frame finished?"
        # "Build sum of many FFT frames, point by point."
        n294 = xnode ("FFT")("real data in"=w369, "reset"=w368, "imaginary data in"=fxp<+/-,16,1> 0.0) -> ("data index"=w361:u16, "real data out"=w347:fxp<+/-,30,15>)  [unwired: 1 out]
        n295 = To Unsigned Long Integer(number=w361) -> (unsigned 32bit integer=w353:u32)
        n296 = xnode ("Memory Method Node")("Address"=w353, "Memory In"=w350) -> ("Data"=w352:fxp<+/-,27,12>, "Memory Out"=w349:refnum<k21>)
        n297 = feedback #94() -> (w363:u16)  [unwired: 1 in]
        n298 = feedback-in #94(w361) -> ()
        n299 = xnode ("High Throughput Multiply")("x"=w347, "y"=w347) -> ("x*y"=w346:fxp<+/-,60,30>)
        n300 = Build Array(w361, w363) -> (→"SuccessiveIndeces":u16[])
        n301 = To Fixed-Point(fixed-point type=fxp<+/-,27,12> 0.0 ("Data"), number=w346) -> (fixed-point=w344:fxp<+/-,27,12>)
        n302 = xnode ("High Throughput Add")("x"=w352, "y"=w344) -> ("x+y"=w351:fxp<+/-,28,13>)  [unwired: 1 out]
        n303 = To Fixed-Point(fixed-point type=fxp<+/-,27,12> 0.0 ("Data"), number=w351) -> (fixed-point=w354:fxp<+/-,27,12>)
        n304 = Greater Or Equal?(x=w361, y=u16 8191) -> (x >= y?=w356:bool)
        n305 = xnode ("Memory Method Node")("Address"=w353, "Data"=w354, "Memory In"=w349) -> ("Memory Out"=w348:refnum<k21>)
        n306 = feedback #95(FALSE) -> (w359:bool)
        n307 = call-poly <instrlib>:"Count Up.vi"("increment"=w356, "reset"=w359) -> ("count out"=w358:u16)  [unwired: 13 in]
        n308 = Greater Or Equal?(x=w358, y="#Avg") -> (x >= y?=w366:bool)
        n309 = feedback-in #95(w366) -> ()
        n310 = case shown="True" w366 {
          tunnel: w348 -> [_ w389]
          frame False {
          }
          frame True {
            n311 = for {
              N: 8192 ("dimension size") -> [_]
              tunnel: w389 -> [w391]
              i -> [w394]
              # "Transfer summed collection of frames to host."
              # "Reset to zeros"
              n312 = To Unsigned Long Integer(number=w394) -> (unsigned 32bit integer=w396:u32)
              n313 = xnode ("Memory Method Node")("Address"=w396, "Memory In"=w391) -> ("Data"=w395:fxp<+/-,27,12>, "Memory Out"=w392:refnum<k21>)
              n314 = Integer to Fixed-Point Cast(fixed-point type=fxp<+/-,30,15> 0.0 ("real data out"), integer=w394) -> (fixed-point=w399:fxp<+/-,30,15>)
              n315 = Build Array(w399, w395) -> (w397:fxp<+/-,30,15>[])
              n316 = xnode ("Memory Method Node")("Address"=w396, "Data"=fxp<+/-,27,12> 0.0, "Memory In"=w392) -> ()  [unwired: 1 out]
              n317 = xnode ("FIFO Method Node")("Element"=w397, "Timeout"=0) -> ()  [unwired: 1 in, 2 out]
            }
          }
        }
      }
      frame True {
      }
    }
    "NoiseFloorFFT_LoopCount" <- w340
  }
  n318 = while {
    shift-right: [w404] -> _
    shift-left: TRUE -> [w405]
    tunnel: w4 -> [w402]
    i -> [w406]
    stop <- FALSE stop-if-true
    # "Most recent processed point"
    # "Noise Floor FFT"
    n319 = xnode ("FIFO Method Node")("Timeout"=0) -> ("Element"=w408:fxp<+/-,16,1>, "Timed Out?"=w403:bool)  [unwired: 1 in, 1 out]
    "ReceiverTimed Out 2" <- w403
    n320 = case shown="False" w403 {
      tunnel: w408 -> [w435 _]
      tunnel: w405 -> [w434 w467]
      tunnel: [FALSE w467] -> w404
      tunnel: w402 -> [w416 _]
      frame False {
        # "Is collection of frames finished?"
        # "Is frame finished?"
        # "Build sum of many FFT frames, point by point."
        n321 = xnode ("FFT 2")("real data in"=w435, "reset"=w434, "imaginary data in"=fxp<+/-,16,1> 0.0) -> ("data index"=w427:u16, "real data out"=w411:fxp<+/-,30,15>)  [unwired: 1 out]
        n322 = To Unsigned Long Integer(number=w427) -> (unsigned 32bit integer=w419:u32)
        n323 = xnode ("Memory Method Node")("Address"=w419, "Memory In"=w416) -> ("Data"=w418:fxp<+/-,27,12>, "Memory Out"=w415:refnum<k21>)
        n324 = feedback #96() -> (w429:u16)  [unwired: 1 in]
        n325 = feedback-in #96(w427) -> ()
        n326 = xnode ("High Throughput Multiply")("x"=w411, "y"=w411) -> ("x*y"=w413:fxp<+/-,60,30>)
        n327 = Build Array(w427, w429) -> (→"SuccessiveIndeces 2":u16[])
        n328 = To Fixed-Point(fixed-point type=fxp<+/-,27,12> 0.0 ("Data"), number=w413) -> (fixed-point=w410:fxp<+/-,27,12>)
        n329 = xnode ("High Throughput Add")("x"=w418, "y"=w410) -> ("x+y"=w417:fxp<+/-,28,13>)  [unwired: 1 out]
        n330 = To Fixed-Point(fixed-point type=fxp<+/-,27,12> 0.0 ("Data"), number=w417) -> (fixed-point=w420:fxp<+/-,27,12>)
        n331 = Greater Or Equal?(x=w427, y=u16 8191) -> (x >= y?=w422:bool)
        n332 = xnode ("Memory Method Node")("Address"=w419, "Data"=w420, "Memory In"=w415) -> ("Memory Out"=w414:refnum<k21>)
        n333 = feedback #97(FALSE) -> (w425:bool)
        n334 = call-poly <instrlib>:"Count Up.vi"("increment"=w422, "reset"=w425) -> ("count out"=w424:u16)  [unwired: 13 in]
        n335 = Greater Or Equal?(x=w424, y="#Avg 2") -> (x >= y?=w432:bool)
        n336 = feedback-in #97(w432) -> ()
        n337 = case shown="True" w432 {
          tunnel: w414 -> [_ w455]
          frame False {
          }
          frame True {
            n338 = for {
              N: 8192 ("dimension size") -> [_]
              tunnel: w455 -> [w457]
              i -> [w460]
              # "Transfer summed collection of frames to host."
              # "Reset to zeros"
              n339 = To Unsigned Long Integer(number=w460) -> (unsigned 32bit integer=w462:u32)
              n340 = xnode ("Memory Method Node")("Address"=w462, "Memory In"=w457) -> ("Data"=w461:fxp<+/-,27,12>, "Memory Out"=w458:refnum<k21>)
              n341 = Integer to Fixed-Point Cast(fixed-point type=fxp<+/-,30,15> 0.0 ("real data out"), integer=w460) -> (fixed-point=w465:fxp<+/-,30,15>)
              n342 = Build Array(w465, w461) -> (w463:fxp<+/-,30,15>[])
              n343 = xnode ("Memory Method Node")("Address"=w462, "Data"=fxp<+/-,27,12> 0.0, "Memory In"=w458) -> ()  [unwired: 1 out]
              n344 = xnode ("FIFO Method Node")("Element"=w463, "Timeout"=0) -> ()  [unwired: 1 in, 2 out]
            }
          }
        }
      }
      frame True {
      }
    }
    "NoiseFloorFFT_LoopCount 2" <- w406
  }
  n345 = node-c288(w11) -> ()
